vi "OP500ZP_CLUSTER_SOFTS.vi"(10 "MESURES":T1, 11 "EmptyTab":string[][](array[string])) -> (4 "Tab1":string[][](array[string]), 6 "PASS/FAIL":bool[](array[boolean]))   [LabVIEW 2020]
uses:
  VG/PackType.vi
  VG/IS30%.vi
panel:
  out "errout":errorcluster caption="error out"
  in  "errin":errorcluster
  out "VG IS30% ?":bool
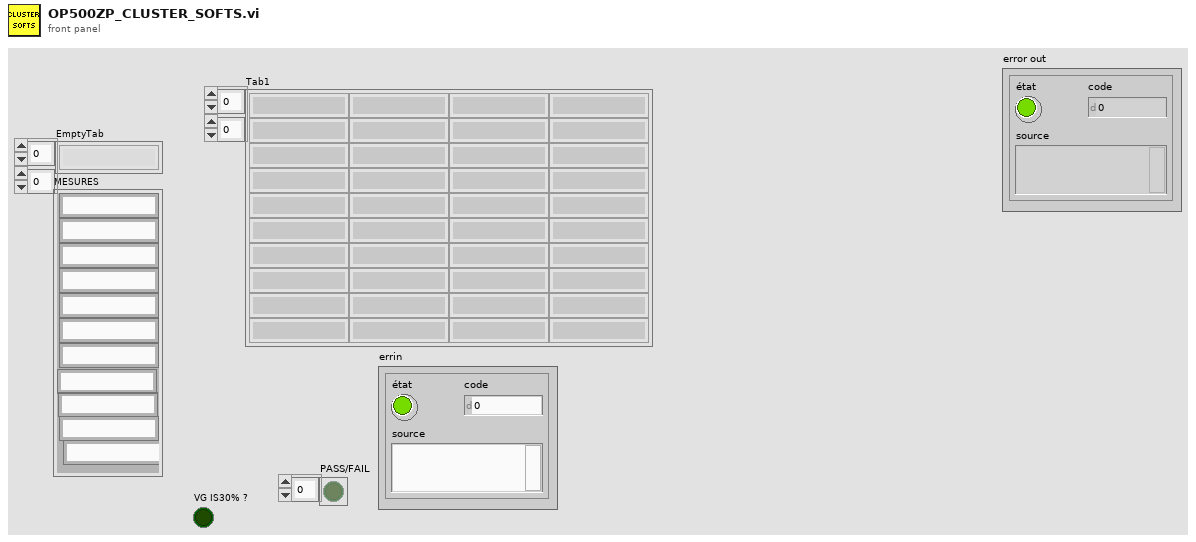
[diagram p1: front panel]
types:
  T1 = cluster{string, string, string, string, string, string, string, string, string, string, string}
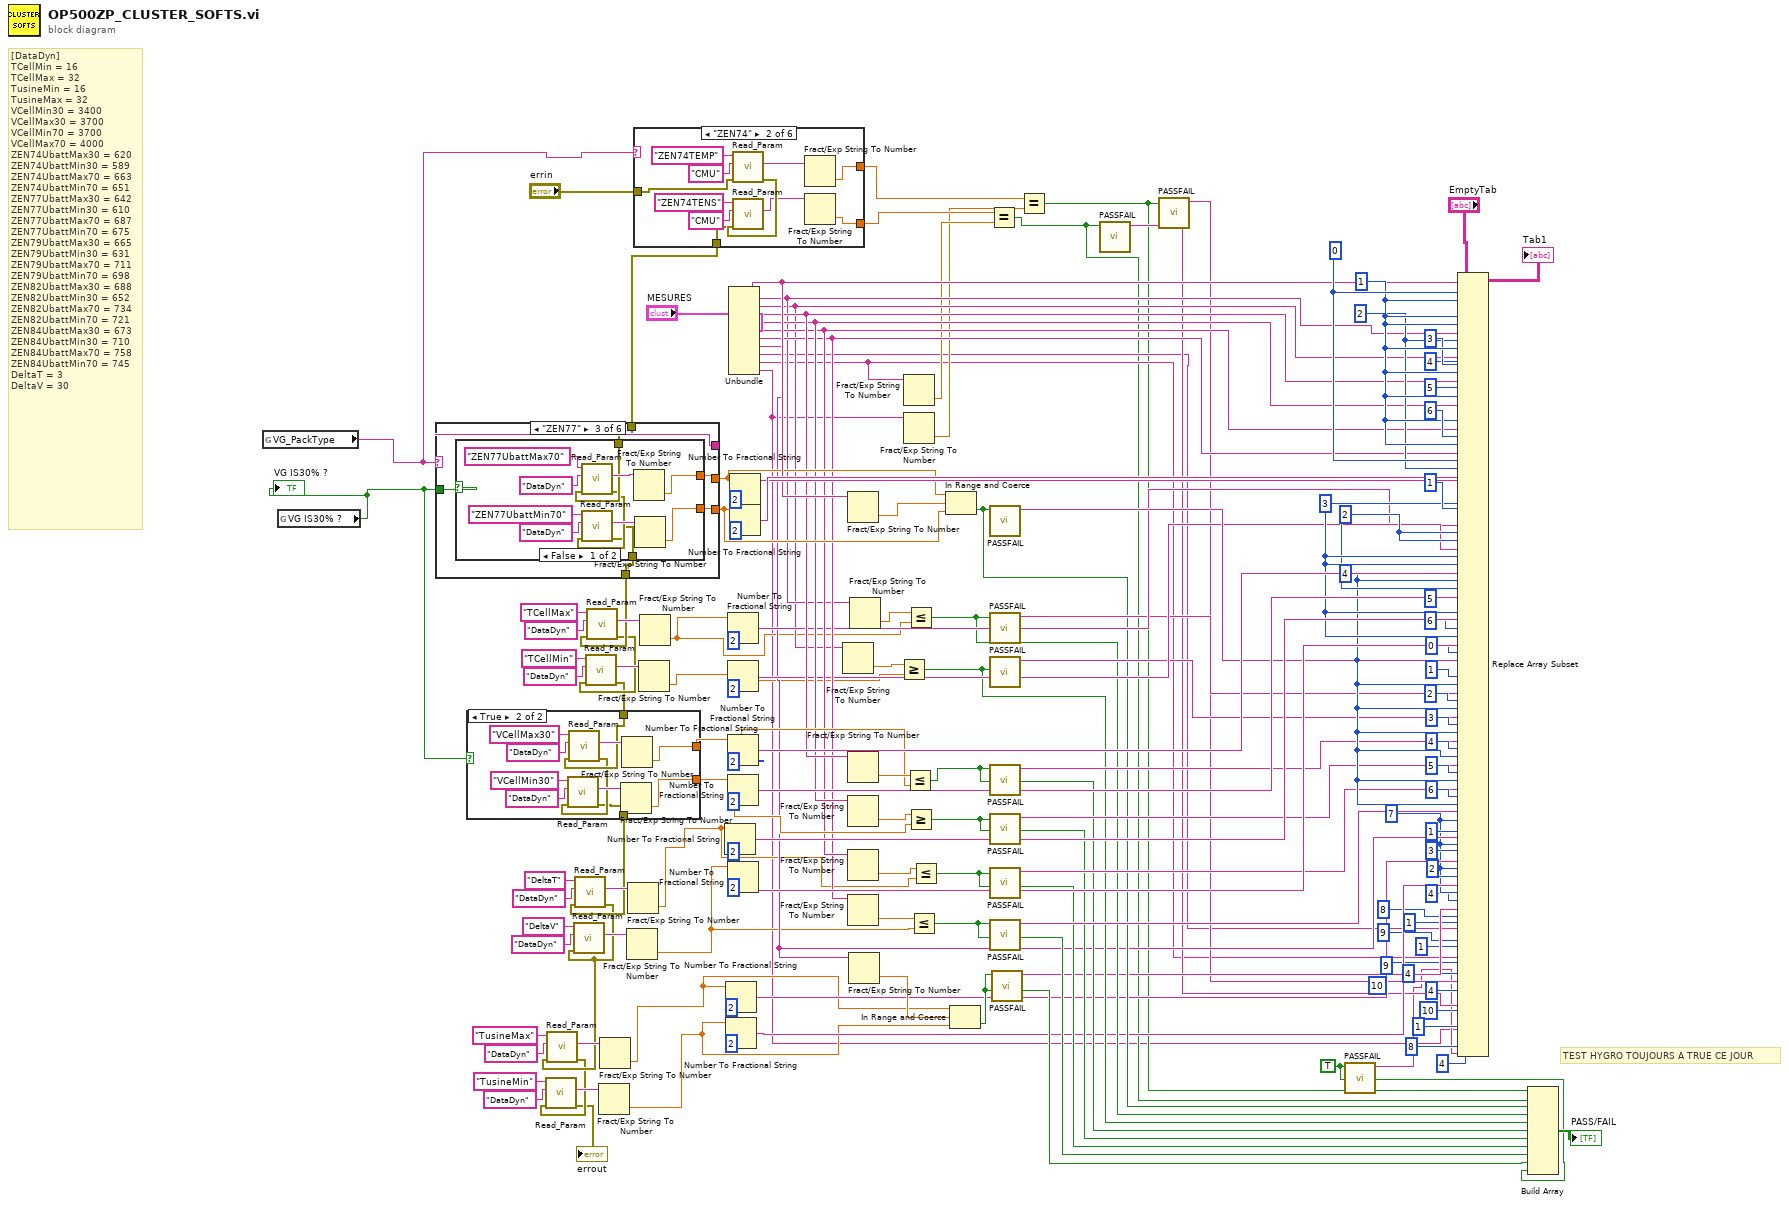
[diagram p0: block diagram]
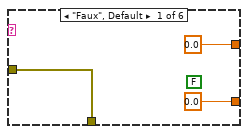
[diagram p2: hidden frame]
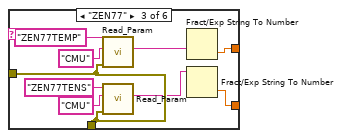
[diagram p3: hidden frame]
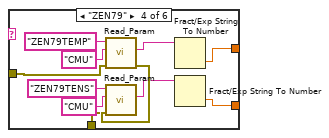
[diagram p4: hidden frame]
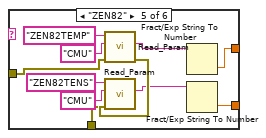
[diagram p5: hidden frame]
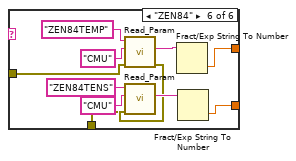
[diagram p6: hidden frame]
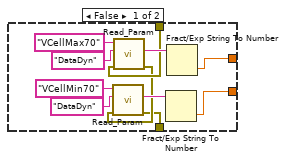
[diagram p7: hidden frame]
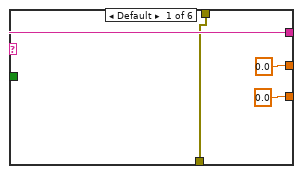
[diagram p8: hidden frame]
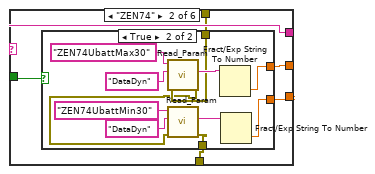
[diagram p9: hidden frame]
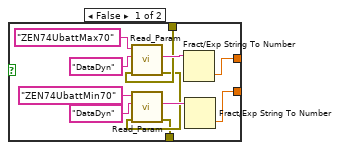
[diagram p10: hidden frame]
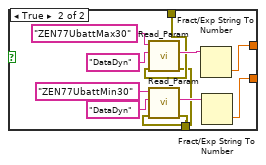
[diagram p11: hidden frame]
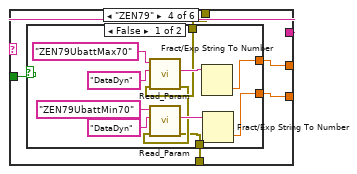
[diagram p12: hidden frame]
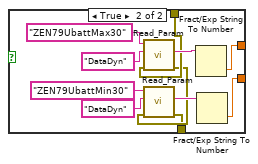
[diagram p13: hidden frame]
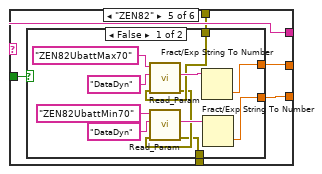
[diagram p14: hidden frame]
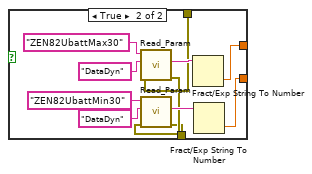
[diagram p15: hidden frame]
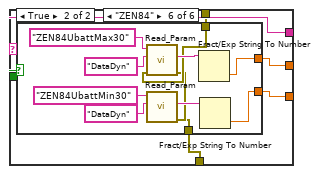
[diagram p16: hidden frame]
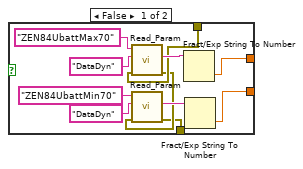
[diagram p17: hidden frame]
diagram:
  w2 = TRUE ("E")
  w61 = 7 ("indice (ligne)")
  w116 = 2 ("indice désactivé (ligne)")
  w88 = 4 ("indice (ligne)")
  w117 = 3 ("indice désactivé (col)")
  w130 = 2 ("indice désactivé (ligne)")
  w137 = 1 ("indice (col)")
  w140 = 0 ("indice (ligne)")
  # "TEST HYGRO TOUJOURS A TRUE CE JOUR"
  # "[DataDyn]\nTCellMin = 16\nTCellMax = 32\nTusineMin = 16\nTusineMax = 32\nVCellMin30 = 3400\nVCellMax30 = 3700\nVCellMin70 = 3700\nVCellMax70 = 4000\nZEN74UbattMax30 = 620\nZEN74UbattMin30 = 589\nZEN74UbattMax70 = 663\nZEN74UbattMin70 = 651\nZEN77UbattMax30 = 642\nZEN77UbattMin30 = 610\nZEN77UbattMax70 = 687\nZEN77UbattMin70 = 675\nZEN79UbattMax30 = 665\nZEN79UbattMin30 = 631\nZEN79UbattMax70 = 711\nZEN79UbattMin70 = 698\nZEN82UbattMax30 = 688\nZEN82UbattMin30 = 652\nZEN82UbattMax70 = 734\nZEN82UbattMin70 = 721\nZEN84UbattMax30 = 673\nZEN84UbattMin30 = 710\nZEN84UbattMax70 = 758\nZEN84UbattMin70 = 745\nDeltaT = 3\nDeltaV = 30"
  n1 = global read "PackType.vi" "VG_PackType"() -> (w8:string)
  n2 = global read "IS30%.vi" "VG IS30% ?"() -> (w129:bool)
  "VG IS30% ?" <- w129
  n3 = case shown="\"ZEN74\"" w8 {
    tunnel: [0.0 ("ZEN84TEMP") w151 w162 w170 w181 w195] -> w55
    tunnel: [0.0 ("ZEN84TENS") w149 w160 w169 w180 w194] -> w54
    tunnel: "errin" -> [w146 w155 w164 w175 w186 w193]
    tunnel: [w146 w153 w164 w173 w184 w191] -> w16
    frame "Faux", Default {
      (unwired) FALSE
    }
    frame "ZEN74" {
      n4 = call <userlib>:"Read_Param.vi"("errin"=w155, "section"="CMU", "key"="ZEN74TEMP") -> ("error out"=w154:errorcluster, "str"=w152:string)  [unwired: 4 in, 3 out]
      n5 = call <userlib>:"Read_Param.vi"("errin"=w154, "section"="CMU", "key"="ZEN74TENS") -> ("error out"=w153:errorcluster, "str"=w150:string)  [unwired: 4 in, 3 out]
      n6 = Fract/Exp String To Number(string=w152) -> (number=w151:dbl)  [unwired: 3 in, 1 out]
      n7 = Fract/Exp String To Number(string=w150) -> (number=w149:dbl)  [unwired: 3 in, 1 out]
    }
    frame "ZEN77" {
      n8 = call <userlib>:"Read_Param.vi"("errin"=w164, "section"="CMU", "key"="ZEN77TEMP") -> ("str"=w163:string)  [unwired: 4 in, 4 out]
      n9 = call <userlib>:"Read_Param.vi"("errin"=w164, "section"="CMU", "key"="ZEN77TENS") -> ("str"=w161:string)  [unwired: 4 in, 4 out]
      n10 = Fract/Exp String To Number(string=w163) -> (number=w162:dbl)  [unwired: 3 in, 1 out]
      n11 = Fract/Exp String To Number(string=w161) -> (number=w160:dbl)  [unwired: 3 in, 1 out]
    }
    frame "ZEN79" {
      n12 = call <userlib>:"Read_Param.vi"("errin"=w175, "section"="CMU", "key"="ZEN79TEMP") -> ("error out"=w174:errorcluster, "str"=w172:string)  [unwired: 4 in, 3 out]
      n13 = call <userlib>:"Read_Param.vi"("errin"=w174, "section"="CMU", "key"="ZEN79TENS") -> ("error out"=w173:errorcluster, "str"=w171:string)  [unwired: 4 in, 3 out]
      n14 = Fract/Exp String To Number(string=w172) -> (number=w170:dbl)  [unwired: 3 in, 1 out]
      n15 = Fract/Exp String To Number(string=w171) -> (number=w169:dbl)  [unwired: 3 in, 1 out]
    }
    frame "ZEN82" {
      n16 = call <userlib>:"Read_Param.vi"("errin"=w186, "section"="CMU", "key"="ZEN82TEMP") -> ("error out"=w185:errorcluster, "str"=w183:string)  [unwired: 4 in, 3 out]
      n17 = call <userlib>:"Read_Param.vi"("errin"=w185, "section"="CMU", "key"="ZEN82TENS") -> ("error out"=w184:errorcluster, "str"=w182:string)  [unwired: 4 in, 3 out]
      n18 = Fract/Exp String To Number(string=w183) -> (number=w181:dbl)  [unwired: 3 in, 1 out]
      n19 = Fract/Exp String To Number(string=w182) -> (number=w180:dbl)  [unwired: 3 in, 1 out]
    }
    frame "ZEN84" {
      n20 = call <userlib>:"Read_Param.vi"("errin"=w193, "section"="CMU", "key"="ZEN84TEMP") -> ("error out"=w192:errorcluster, "str"=w197:string)  [unwired: 4 in, 3 out]
      n21 = call <userlib>:"Read_Param.vi"("errin"=w192, "section"="CMU", "key"="ZEN84TENS") -> ("error out"=w191:errorcluster, "str"=w196:string)  [unwired: 4 in, 3 out]
      n22 = Fract/Exp String To Number(string=w197) -> (number=w195:dbl)  [unwired: 3 in, 1 out]
      n23 = Fract/Exp String To Number(string=w196) -> (number=w194:dbl)  [unwired: 3 in, 1 out]
    }
  }
  n24 = case shown="\"ZEN77\"" w8 {
    selector: w8 -> [w205 w208 w236 w264 w292 w320]
    tunnel: [0.0 ("ZEN84UbattMax30") w211 w239 w267 w295 w323] -> w113
    tunnel: [0.0 ("ZEN84UbattMin30") w210 w238 w266 w294 w322] -> w112
    tunnel: w129 -> [_ w209 w237 w265 w293 w321]
    tunnel: [w205 w208 w236 w264 w292 w320] -> _
    tunnel: w16 -> [w202 w207 w235 w263 w291 w319]
    tunnel: [w202 w206 w234 w262 w290 w318] -> w15
    frame Default {
    }
    frame "ZEN74" {
      n25 = case shown="True" w209 {
        tunnel: [w216 w227] -> w211
        tunnel: [w215 w226] -> w210
        tunnel: w207 -> [w214 w225]
        tunnel: [w212 w223] -> w206
        frame False {
          n26 = call <userlib>:"Read_Param.vi"("errin"=w214, "section"="DataDyn", "key"="ZEN74UbattMax70") -> ("error out"=w213:errorcluster, "str"=w220:string)  [unwired: 4 in, 3 out]
          n27 = call <userlib>:"Read_Param.vi"("errin"=w213, "section"="DataDyn", "key"="ZEN74UbattMin70") -> ("error out"=w212:errorcluster, "str"=w219:string)  [unwired: 4 in, 3 out]
          n28 = Fract/Exp String To Number(string=w220) -> (number=w216:dbl)  [unwired: 3 in, 1 out]
          n29 = Fract/Exp String To Number(string=w219) -> (number=w215:dbl)  [unwired: 3 in, 1 out]
        }
        frame True {
          n30 = call <userlib>:"Read_Param.vi"("errin"=w225, "section"="DataDyn", "key"="ZEN74UbattMax30") -> ("error out"=w224:errorcluster, "str"=w231:string)  [unwired: 4 in, 3 out]
          n31 = call <userlib>:"Read_Param.vi"("errin"=w224, "section"="DataDyn", "key"="ZEN74UbattMin30") -> ("error out"=w223:errorcluster, "str"=w230:string)  [unwired: 4 in, 3 out]
          n32 = Fract/Exp String To Number(string=w231) -> (number=w227:dbl)  [unwired: 3 in, 1 out]
          n33 = Fract/Exp String To Number(string=w230) -> (number=w226:dbl)  [unwired: 3 in, 1 out]
        }
      }
    }
    frame "ZEN77" {
      n34 = case shown="False" w237 {
        tunnel: [w244 w255] -> w239
        tunnel: [w243 w254] -> w238
        tunnel: w235 -> [w242 w253]
        tunnel: [w240 w251] -> w234
        frame False {
          n35 = call <userlib>:"Read_Param.vi"("errin"=w242, "section"="DataDyn", "key"="ZEN77UbattMax70") -> ("error out"=w241:errorcluster, "str"=w248:string)  [unwired: 4 in, 3 out]
          n36 = call <userlib>:"Read_Param.vi"("errin"=w241, "section"="DataDyn", "key"="ZEN77UbattMin70") -> ("error out"=w240:errorcluster, "str"=w247:string)  [unwired: 4 in, 3 out]
          n37 = Fract/Exp String To Number(string=w248) -> (number=w244:dbl)  [unwired: 3 in, 1 out]
          n38 = Fract/Exp String To Number(string=w247) -> (number=w243:dbl)  [unwired: 3 in, 1 out]
        }
        frame True {
          n39 = call <userlib>:"Read_Param.vi"("errin"=w253, "section"="DataDyn", "key"="ZEN77UbattMax30") -> ("error out"=w252:errorcluster, "str"=w259:string)  [unwired: 4 in, 3 out]
          n40 = call <userlib>:"Read_Param.vi"("errin"=w252, "section"="DataDyn", "key"="ZEN77UbattMin30") -> ("error out"=w251:errorcluster, "str"=w258:string)  [unwired: 4 in, 3 out]
          n41 = Fract/Exp String To Number(string=w259) -> (number=w255:dbl)  [unwired: 3 in, 1 out]
          n42 = Fract/Exp String To Number(string=w258) -> (number=w254:dbl)  [unwired: 3 in, 1 out]
        }
      }
    }
    frame "ZEN79" {
      n43 = case shown="False" w265 {
        tunnel: [w272 w283] -> w267
        tunnel: [w271 w282] -> w266
        tunnel: w263 -> [w270 w281]
        tunnel: [w268 w279] -> w262
        frame False {
          n44 = call <userlib>:"Read_Param.vi"("errin"=w270, "section"="DataDyn", "key"="ZEN79UbattMax70") -> ("error out"=w269:errorcluster, "str"=w276:string)  [unwired: 4 in, 3 out]
          n45 = call <userlib>:"Read_Param.vi"("errin"=w269, "section"="DataDyn", "key"="ZEN79UbattMin70") -> ("error out"=w268:errorcluster, "str"=w275:string)  [unwired: 4 in, 3 out]
          n46 = Fract/Exp String To Number(string=w276) -> (number=w272:dbl)  [unwired: 3 in, 1 out]
          n47 = Fract/Exp String To Number(string=w275) -> (number=w271:dbl)  [unwired: 3 in, 1 out]
        }
        frame True {
          n48 = call <userlib>:"Read_Param.vi"("errin"=w281, "section"="DataDyn", "key"="ZEN79UbattMax30") -> ("error out"=w280:errorcluster, "str"=w287:string)  [unwired: 4 in, 3 out]
          n49 = call <userlib>:"Read_Param.vi"("errin"=w280, "section"="DataDyn", "key"="ZEN79UbattMin30") -> ("error out"=w279:errorcluster, "str"=w286:string)  [unwired: 4 in, 3 out]
          n50 = Fract/Exp String To Number(string=w287) -> (number=w283:dbl)  [unwired: 3 in, 1 out]
          n51 = Fract/Exp String To Number(string=w286) -> (number=w282:dbl)  [unwired: 3 in, 1 out]
        }
      }
    }
    frame "ZEN82" {
      n52 = case shown="False" w293 {
        tunnel: [w300 w311] -> w295
        tunnel: [w299 w310] -> w294
        tunnel: w291 -> [w298 w309]
        tunnel: [w296 w307] -> w290
        frame False {
          n53 = call <userlib>:"Read_Param.vi"("errin"=w298, "section"="DataDyn", "key"="ZEN82UbattMax70") -> ("error out"=w297:errorcluster, "str"=w304:string)  [unwired: 4 in, 3 out]
          n54 = call <userlib>:"Read_Param.vi"("errin"=w297, "section"="DataDyn", "key"="ZEN82UbattMin70") -> ("error out"=w296:errorcluster, "str"=w303:string)  [unwired: 4 in, 3 out]
          n55 = Fract/Exp String To Number(string=w304) -> (number=w300:dbl)  [unwired: 3 in, 1 out]
          n56 = Fract/Exp String To Number(string=w303) -> (number=w299:dbl)  [unwired: 3 in, 1 out]
        }
        frame True {
          n57 = call <userlib>:"Read_Param.vi"("errin"=w309, "section"="DataDyn", "key"="ZEN82UbattMax30") -> ("error out"=w308:errorcluster, "str"=w315:string)  [unwired: 4 in, 3 out]
          n58 = call <userlib>:"Read_Param.vi"("errin"=w308, "section"="DataDyn", "key"="ZEN82UbattMin30") -> ("error out"=w307:errorcluster, "str"=w314:string)  [unwired: 4 in, 3 out]
          n59 = Fract/Exp String To Number(string=w315) -> (number=w311:dbl)  [unwired: 3 in, 1 out]
          n60 = Fract/Exp String To Number(string=w314) -> (number=w310:dbl)  [unwired: 3 in, 1 out]
        }
      }
    }
    frame "ZEN84" {
      n61 = case shown="True" w321 {
        tunnel: [w327 w339] -> w323
        tunnel: [w328 w338] -> w322
        tunnel: w319 -> [w326 w337]
        tunnel: [w324 w335] -> w318
        frame False {
          n62 = call <userlib>:"Read_Param.vi"("errin"=w326, "section"="DataDyn", "key"="ZEN84UbattMax70") -> ("error out"=w325:errorcluster, "str"=w330:string)  [unwired: 4 in, 3 out]
          n63 = call <userlib>:"Read_Param.vi"("errin"=w325, "section"="DataDyn", "key"="ZEN84UbattMin70") -> ("error out"=w324:errorcluster, "str"=w329:string)  [unwired: 4 in, 3 out]
          n64 = Fract/Exp String To Number(string=w330) -> (number=w327:dbl)  [unwired: 3 in, 1 out]
          n65 = Fract/Exp String To Number(string=w329) -> (number=w328:dbl)  [unwired: 3 in, 1 out]
        }
        frame True {
          n66 = call <userlib>:"Read_Param.vi"("errin"=w337, "section"="DataDyn", "key"="ZEN84UbattMax30") -> ("error out"=w336:errorcluster, "str"=w342:string)  [unwired: 4 in, 3 out]
          n67 = call <userlib>:"Read_Param.vi"("errin"=w336, "section"="DataDyn", "key"="ZEN84UbattMin30") -> ("error out"=w335:errorcluster, "str"=w341:string)  [unwired: 4 in, 3 out]
          n68 = Fract/Exp String To Number(string=w342) -> (number=w339:dbl)  [unwired: 3 in, 1 out]
          n69 = Fract/Exp String To Number(string=w341) -> (number=w338:dbl)  [unwired: 3 in, 1 out]
        }
      }
    }
  }
  n70 = call <userlib>:"Read_Param.vi"("errin"=w15, "section"="DataDyn", "key"="TCellMax") -> ("error out"=w14:errorcluster, "str"=w39:string)  [unwired: 4 in, 3 out]
  n71 = call <userlib>:"Read_Param.vi"("errin"=w14, "section"="DataDyn", "key"="TCellMin") -> ("error out"=w13:errorcluster, "str"=w35:string)  [unwired: 4 in, 3 out]
  n72 = case shown="True" w129 {
    tunnel: [w350 w362] -> w110
    tunnel: [w349 w361] -> w106
    tunnel: w13 -> [w348 w359]
    tunnel: [w346 w357] -> w12
    frame False {
      n73 = call <userlib>:"Read_Param.vi"("errin"=w348, "section"="DataDyn", "key"="VCellMax70") -> ("error out"=w347:errorcluster, "str"=w354:string)  [unwired: 4 in, 3 out]
      n74 = call <userlib>:"Read_Param.vi"("errin"=w347, "section"="DataDyn", "key"="VCellMin70") -> ("error out"=w346:errorcluster, "str"=w351:string)  [unwired: 4 in, 3 out]
      n75 = Fract/Exp String To Number(string=w351) -> (number=w349:dbl)  [unwired: 3 in, 1 out]
      n76 = Fract/Exp String To Number(string=w354) -> (number=w350:dbl)  [unwired: 3 in, 1 out]
    }
    frame True {
      n77 = call <userlib>:"Read_Param.vi"("errin"=w359, "section"="DataDyn", "key"="VCellMax30") -> ("error out"=w358:errorcluster, "str"=w366:string)  [unwired: 4 in, 3 out]
      n78 = call <userlib>:"Read_Param.vi"("errin"=w358, "section"="DataDyn", "key"="VCellMin30") -> ("error out"=w357:errorcluster, "str"=w363:string)  [unwired: 4 in, 3 out]
      n79 = Fract/Exp String To Number(string=w363) -> (number=w361:dbl)  [unwired: 3 in, 1 out]
      n80 = Fract/Exp String To Number(string=w366) -> (number=w362:dbl)  [unwired: 3 in, 1 out]
    }
  }
  n81 = call <userlib>:"Read_Param.vi"("errin"=w12, "section"="DataDyn", "key"="DeltaT") -> ("error out"=w11:errorcluster, "str"=w32:string)  [unwired: 4 in, 3 out]
  n82 = call <userlib>:"Read_Param.vi"("errin"=w11, "section"="DataDyn", "key"="TusineMax") -> ("error out"=w10:errorcluster, "str"=w24:string)  [unwired: 4 in, 3 out]
  n83 = call <userlib>:"Read_Param.vi"("errin"=w10, "section"="DataDyn", "key"="TusineMin") -> ("error out"=→"errout":errorcluster, "str"=w21:string)  [unwired: 4 in, 3 out]
  n84 = call <userlib>:"Read_Param.vi"("errin"=w11, "section"="DataDyn", "key"="DeltaV") -> ("str"=w29:string)  [unwired: 4 in, 4 out]
  n85 = Fract/Exp String To Number(string=w21) -> (number=w18:dbl)  [unwired: 3 in, 1 out]
  n86 = Fract/Exp String To Number(string=w24) -> (number=w19:dbl)  [unwired: 3 in, 1 out]
  n87 = Fract/Exp String To Number(string=w29) -> (number=w26:dbl)  [unwired: 3 in, 1 out]
  n88 = Fract/Exp String To Number(string=w32) -> (number=w27:dbl)  [unwired: 3 in, 1 out]
  n89 = Fract/Exp String To Number(string=w35) -> (number=w34:dbl)  [unwired: 3 in, 1 out]
  n90 = Fract/Exp String To Number(string=w39) -> (number=w38:dbl)  [unwired: 3 in, 1 out]
  n91 = Number To Fractional String(number=w27, precision (6)=i16 2 ("précision (6)")) -> (F-format string=w121:string)  [unwired: 2 in]
  n92 = Number To Fractional String(number=w19, precision (6)=i16 2 ("précision (6)")) -> (F-format string=w66:string)  [unwired: 2 in]
  n93 = Number To Fractional String(number=w18, precision (6)=i16 2 ("précision (6)")) -> (F-format string=w65:string)  [unwired: 2 in]
  n94 = Number To Fractional String(number=w38, precision (6)=i16 2 ("précision (6)")) -> (F-format string=w91:string)  [unwired: 2 in]
  n95 = Number To Fractional String(number=w34, precision (6)=i16 2 ("précision (6)")) -> (F-format string=w92:string)  [unwired: 2 in]
  n96 = Number To Fractional String(number=w110, precision (6)=i16 2 ("précision (6)")) -> (F-format string=w126:string)  [unwired: 2 in]
  n97 = Number To Fractional String(number=w106, precision (6)=i16 2 ("précision (6)")) -> (F-format string=w124:string)  [unwired: 2 in]
  n98 = Number To Fractional String(number=w26, precision (6)=i16 2 ("précision (6)")) -> (F-format string=w120:string)  [unwired: 2 in]
  n99 = Unbundle("MESURES") -> (w115:string, w81:string, w80:string, w109:string, w107:string, w104:string, w103:string, w70:string, w45:string, w44:string, w1:string)
  n100 = Number To Fractional String(number=w113, precision (6)=i16 2 ("précision (6)")) -> (F-format string=w138:string)  [unwired: 2 in]
  n101 = Number To Fractional String(number=w112, precision (6)=i16 2 ("précision (6)")) -> (F-format string=w139:string)  [unwired: 2 in]
  n102 = Fract/Exp String To Number(string=w80) -> (number=w101:dbl)  [unwired: 3 in, 1 out]
  n103 = Fract/Exp String To Number(string=w115) -> (number=w114:dbl)  [unwired: 3 in, 1 out]
  n104 = Fract/Exp String To Number(string=w109) -> (number=w111:dbl)  [unwired: 3 in, 1 out]
  n105 = Fract/Exp String To Number(string=w107) -> (number=w108:dbl)  [unwired: 3 in, 1 out]
  n106 = Fract/Exp String To Number(string=w104) -> (number=w79:dbl)  [unwired: 3 in, 1 out]
  n107 = Fract/Exp String To Number(string=w103) -> (number=w105:dbl)  [unwired: 3 in, 1 out]
  n108 = Fract/Exp String To Number(string=w70) -> (number=w68:dbl)  [unwired: 3 in, 1 out]
  n109 = Fract/Exp String To Number(string=w81) -> (number=w102:dbl)  [unwired: 3 in, 1 out]
  n110 = Greater Or Equal?(x=w101, y=w34) -> (x >= y?=w76:bool)
  n111 = Fract/Exp String To Number(string=w44) -> (number=w53:dbl)  [unwired: 3 in, 1 out]
  n112 = Fract/Exp String To Number(string=w1) -> (number=w52:dbl)  [unwired: 3 in, 1 out]
  n113 = Less Or Equal?(x=w111, y=w110) -> (x <= y?=w75:bool)
  n114 = Less Or Equal?(x=w102, y=w38) -> (x <= y?=w77:bool)
  n115 = Greater Or Equal?(x=w108, y=w106) -> (x >= y?=w74:bool)
  n116 = Less Or Equal?(x=w105, y=w26) -> (x <= y?=w72:bool)
  n117 = Less Or Equal?(x=w79, y=w27) -> (x <= y?=w73:bool)
  n118 = In Range and Coerce(upper limit=w113, x=w114, lower limit=w112) -> (In Range?=w78:bool)  [unwired: 1 out]
  n119 = In Range and Coerce(upper limit=w19, x=w68, lower limit=w18) -> (In Range?=w67:bool)  [unwired: 1 out]
  n120 = Equal?(x=w54, y=w53) -> (x = y?=w43:bool)
  n121 = call <userlib>:"PASSFAIL.vi"("E"=w78) -> ("S"=w98:string)  [unwired: 10 in]
  n122 = call <userlib>:"PASSFAIL.vi"("E"=w77) -> ("S"=w87:string)  [unwired: 10 in]
  n123 = call <userlib>:"PASSFAIL.vi"("E"=w76) -> ("S"=w86:string)  [unwired: 10 in]
  n124 = call <userlib>:"PASSFAIL.vi"("E"=w75) -> ("S"=w85:string)  [unwired: 10 in]
  n125 = call <userlib>:"PASSFAIL.vi"("E"=w74) -> ("S"=w84:string)  [unwired: 10 in]
  n126 = call <userlib>:"PASSFAIL.vi"("E"=w73) -> ("S"=w83:string)  [unwired: 10 in]
  n127 = call <userlib>:"PASSFAIL.vi"("E"=w72) -> ("S"=w82:string)  [unwired: 10 in]
  n128 = call <userlib>:"PASSFAIL.vi"("E"=w67) -> ("S"=w62:string)  [unwired: 10 in]
  n129 = Equal?(x=w55, y=w52) -> (x = y?=w42:bool)
  n130 = call <userlib>:"PASSFAIL.vi"("E"=w43) -> ("S"=w50:string)  [unwired: 10 in]
  n131 = call <userlib>:"PASSFAIL.vi"("E"=w42) -> ("S"=w51:string)  [unwired: 10 in]
  n132 = call <userlib>:"PASSFAIL.vi"("E"=w2) -> ("S"=w3:string)  [unwired: 10 in]
  n133 = Replace Array Subset(array="EmptyTab", new element #1=w115, index (row) #1=w140, index (col) #1=w137, new element #2=w81, index (row) #2=w137, index (col) #2=w137, new element #3=w80, index (row) #3=w130, index (col) #3=w137, new element #4=w109, index (row) #4=3 ("indice désactivé (ligne)"), index (col) #4=w137, new element #5=w107, index (row) #5=4 ("indice désactivé (ligne)"), index (col) #5=w137, new element #6=w104, index (row) #6=5 ("indice désactivé (ligne)"), index (col) #6=w137, new element #7=w103, index (row) #7=6 ("indice désactivé (ligne)"), index (col) #7=w137, new element #8=w139, index (row) #8=w140, index (col) #8=w130, new element #9=w138, new element #10=w91, index (row) #10=1 ("indice désactivé (ligne)"), index (col) #10=w117, new element #11=w92, index (row) #11=w116, index (col) #11=w116, new element #12=w126, index (row) #12=w117, index (col) #12=w117, new element #13=w124, index (row) #13=w88, index (col) #13=w116, new element #14=w121, index (row) #14=5 ("indice (ligne)"), index (col) #14=w117, new element #15=w120, index (row) #15=6 ("indice désactivé (ligne)"), index (col) #15=w117, new element #16=w98, index (row) #16=0 ("indice (ligne)"), index (col) #16=w88, new element #17=w87, index (row) #17=1 ("indice (ligne)"), index (col) #17=w88, new element #18=w86, index (row) #18=2 ("indice (ligne)"), index (col) #18=w88, new element #19=w85, index (row) #19=3 ("indice (ligne)"), index (col) #19=w88, new element #20=w84, index (row) #20=4 ("indice (ligne)"), index (col) #20=w88, new element #21=w83, index (row) #21=5 ("indice (ligne)"), index (col) #21=w88, new element #22=w82, index (row) #22=6 ("indice (ligne)"), index (col) #22=w88, new element #23=w70, index (row) #23=w61, index (col) #23=1 ("indice désactivé (col)"), new element #24=w66, index (row) #24=w61, index (col) #24=3 ("indice désactivé (col)"), new element #25=w65, index (row) #25=w61, index (col) #25=2 ("indice désactivé (col)"), new element #26=w62, index (row) #26=w61, index (col) #26=4 ("indice désactivé (col)"), new element #27=w45, index (row) #27=8 ("indice (ligne)"), index (col) #27=1 ("indice désactivé (col)"), new element #28=w44, index (row) #28=9 ("indice (ligne)"), index (col) #28=1 ("indice désactivé (col)"), new element #29=w51, index (row) #29=9 ("indice (ligne)"), index (col) #29=4 ("indice désactivé (col)"), new element #30=w50, index (row) #30=10 ("indice (ligne)"), index (col) #30=4 ("indice désactivé (col)"), new element #31=w1, index (row) #31=10 ("index (row)"), index (col) #31=1 ("disabled index (col)"), new element #32=w3, index (row) #32=8 ("index (row)"), index (col) #32=4 ("disabled index (col)")) -> (→"Tab1":string[][])  [unwired: 2 in]
  n134 = Build Array(w42, w43, w78, w77, w76, w75, w74, w73, w72, w67, w2) -> (→"PASS/FAIL":bool[])
